vi "Create Symbol Map Daemon.vi"(8 "error in (no error)":errorcluster, 11 "TwinCAT ADS in":refnum<class "TwinCAT ADS.lvclass">) -> (0 "error out":errorcluster, 3 "TwinCAT ADS out":refnum<class "TwinCAT ADS.lvclass">)   [LabVIEW 2018, in "TwinCAT ADS.lvclass"]
uses:
  TwinCAT ADS.lvclass
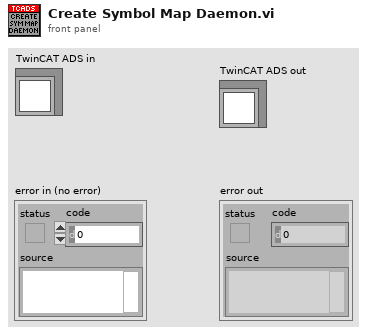
[diagram p1: front panel]
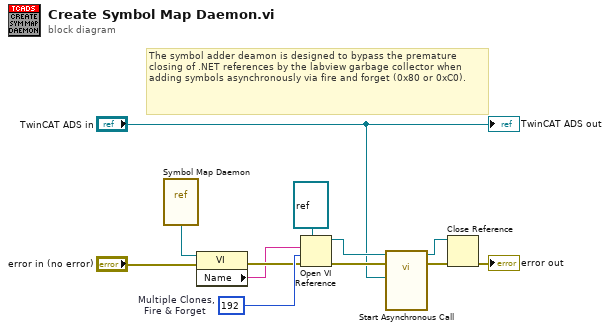
[diagram p0: block diagram]
diagram:
  w12 = 192  # Multiple Clones,   Fire & Forget
  # "The symbol adder deamon is designed to bypass the premature closing of .NET references by the labview garbage collector when adding symbols asynchronously via fire and forget (0x80 or 0xC0)."
  n1 = vi-ref "Symbol Map Daemon.vi"() -> (w2:refnum<vi>)
  n2 = property class="VI"(reference=w2, error in="error in (no error)") -> (error out=w10:errorcluster, "Name"=w9:string)  [unwired: 1 out]
  n3 = Open VI Reference(type specifier VI Refnum (for type only)=refnum<vi> refnum, vi path=w9, options=w12, error in (no error)=w10) -> (vi reference=w7:refnum<vi>, error out=w8:errorcluster)  [unwired: 2 in]
  n4 = call-by-ref "Start Asynchronous Call"(reference=w7, error in=w8, "TwinCAT ADS in"="TwinCAT ADS in") -> (reference out=w5:refnum<vi>, error out=w6:errorcluster)  [unwired: 11 in]
  n5 = Close Reference(reference=w5, error in (no error)=w6) -> (error out=→"error out":errorcluster)
  "TwinCAT ADS out" <- "TwinCAT ADS in"
